vi "Status--Const.vi"() -> (3 "Status Command":string)   [LabVIEW 2017, in "Communications Library.lvlib"]
uses:
  Communications Library.lvlib
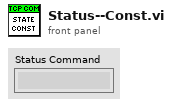
[diagram p1: front panel]
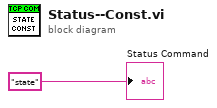
[diagram p0: block diagram]
diagram:
  "Status Command" <- "state" ("data in")
